vi "Wii Out.vi"(4 "error in":errorcluster, 6 "Calibration Data In":T6={"Wiimote 0G Calibration"={"Acceleration X"=127.0, "Acceleration Y"=131.0, "Acceleration Z"=126.0}, "Wiimote 1G Calibration"={"Acceleration X"=127.0, "Acceleration Y"=131.0, "Acceleration Z"=126.0}, "Nunchuk 0G Calibration"={"Acceleration X"=127.0, "Acceleration Y"=131.0, "Acceleration Z"=126.0}, "Nunchuk 1G Calibration"={"Acceleration X"=127.0, "Acceleration Y"=131.0, "Acceleration Z"=126.0}}, 7 "index":i32) -> (0 "error out":errorcluster, 2 "Wii output cluster":T5, 3 "hWiimoteHandle out":u32)   [LabVIEW 2011]
uses:
  Wiimote/Wiimote Buttons.ctl
  Wiimote/Nunchuk Buttons.ctl
  Wiimote/Wiimote Acceleration.ctl
  Wiimote/Wiimote Point.ctl
  Wiimote.lvlib
panel:
  in  "Offset":cluster{"X":dbl, "Y":dbl}={"X"=127.0, "Y"=127.0}
  out "Nunchuk Analog Stick":cluster{dbl, dbl}
  out "Nunchuk Analog Stick":cluster{dbl, dbl}[](graph)
  out "Nunchuk Acceleration":T7(graph)
  out "Wiimote Acceleration":T7(graph)
  out "Nunchuk Buttons":T4
  out "IR Sensor":cluster{"X":u16, "Y":u16}[](graph)
  out "Wiimote Buttons":T3
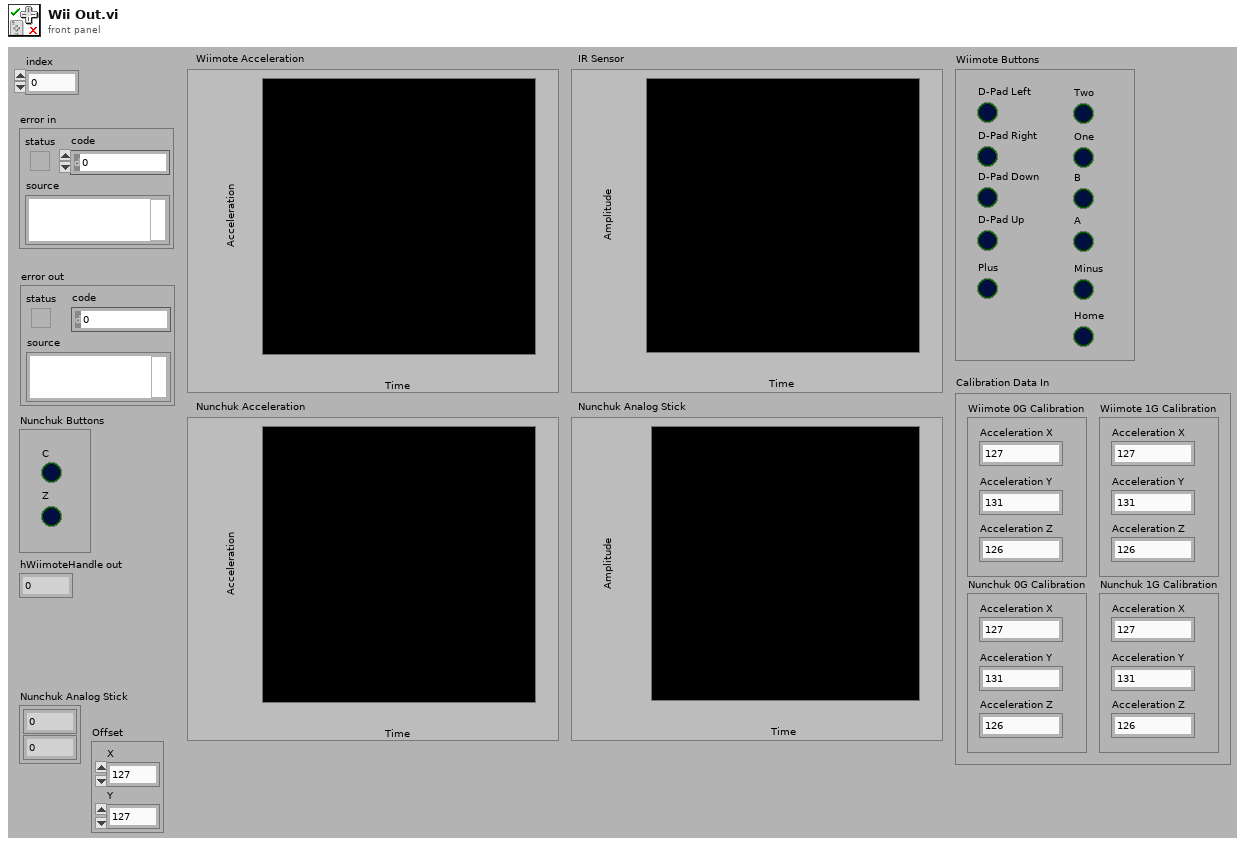
[diagram p1: front panel]
types:
  T1 = typedef "Wiimote.lvlib/Wiimote Acceleration.ctl" = cluster{"Acceleration X":dbl, "Acceleration Y":dbl, "Acceleration Z":dbl}
  T2 = typedef "Wiimote.lvlib/Wiimote Point.ctl" = cluster{"X":u16, "Y":u16}
  T3 = typedef "Wiimote.lvlib/Wiimote Buttons.ctl" = cluster{"D-Pad Left":bool, "D-Pad Right":bool, "D-Pad Down":bool, "D-Pad Up":bool, "Plus":bool, "Two":bool, "One":bool, "B":bool, "A":bool, "Minus":bool, "Home":bool}
  T4 = typedef "Wiimote.lvlib/Nunchuk Buttons.ctl" = cluster{"C":bool, "Z":bool}
  T5 = cluster{"Acceleration Calibrated Out":T1, "Acceleration Calibrated Out":T1, T2[], "Wiimote Buttons":T3, "Nunchuk Buttons":T4, "Nunchuk Analog Stick":cluster{"X":dbl, "Y":dbl}}
  T6 = cluster{"Wiimote 0G Calibration":T1, "Wiimote 1G Calibration":T1, "Nunchuk 0G Calibration":T1, "Nunchuk 1G Calibration":T1}
  T7 = cluster{"Acceleration X":dbl, "Acceleration Y":dbl, "Acceleration Z":dbl}
  T8 = typedef "Wiimote.lvlib/Wiimote IR Sensor.ctl" = cluster{"Point 1":T2, "Point 2":T2, "Point 3":T2, "Point 4":T2}
  T9 = cluster{"Wiimote Buttons":T3, "Wiimote Acceleration Raw":T1, "Wiimote IR Sensor":T8, "Nunchuk Analog Stick":T2, "Nunchuk Acceleration Raw":T1, "Nunchuk Buttons":T4}
  T10 = cluster{"Acceleration Calibrated Out":T1, "Acceleration Calibrated Out":T1, T2[], "Wiimote Buttons":T3, "Nunchuk Buttons":T4, cluster{"X":dbl, "Y":dbl}}
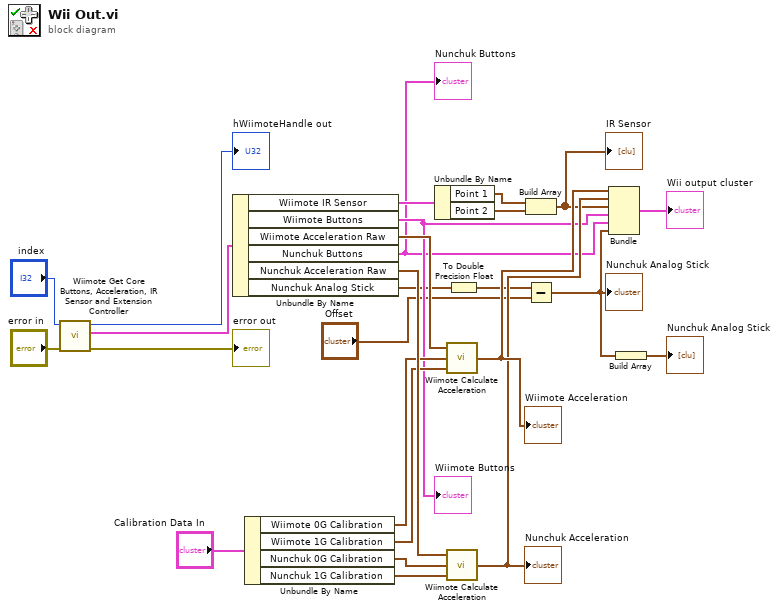
[diagram p0: block diagram]
diagram:
  n1 = call "Wiimote Get Core Buttons, Acceleration, IR Sensor and Extension Controller.vi"("error in"="error in", "hWiimoteHandle in"="index") -> ("error out"=→"error out":errorcluster, "Data out"=w21:T9, "hWiimoteHandle out"=→"hWiimoteHandle out":u32)  [unwired: 7 in]
  n2 = Unbundle By Name(w21) -> ("Wiimote IR Sensor"=w20:T8, "Wiimote Buttons"=w7:T3, "Wiimote Acceleration Raw"=w18:T1, "Nunchuk Buttons"=w6:T4, "Nunchuk Acceleration Raw"=w17:T1, "Nunchuk Analog Stick"=w5:T2)
  "Wiimote Buttons" <- w7
  "Nunchuk Buttons" <- w6
  n3 = Unbundle By Name("Calibration Data In") -> ("Wiimote 0G Calibration"=w13:T1, "Wiimote 1G Calibration"=w14:T1, "Nunchuk 0G Calibration"=w15:T1, "Nunchuk 1G Calibration"=w16:T1)
  n4 = Unbundle By Name(w20) -> ("Point 1"=w23:T2, "Point 2"=w22:T2)
  n5 = call "Wiimote Calculate Acceleration.vi"("Acceleration 1G Calibration"=w14, "Acceleration 0G Calibration"=w13, "Acceleration Raw in"=w18) -> ("Acceleration Calibrated Out"=w10:T1)
  "Wiimote Acceleration" <- w10
  n6 = call "Wiimote Calculate Acceleration.vi"("Acceleration 1G Calibration"=w16, "Acceleration 0G Calibration"=w15, "Acceleration Raw in"=w17) -> ("Acceleration Calibrated Out"=w9:T1)
  "Nunchuk Acceleration" <- w9
  n7 = To Double Precision Float(number=w5) -> (double precision float=w4:cluster{"X":dbl, "Y":dbl})
  n8 = Build Array(w23, w22) -> (w8:T2[])
  "IR Sensor" <- w8
  n9 = Subtract(x=w4, y="Offset") -> (x-y=w2:cluster{"X":dbl, "Y":dbl})
  "Nunchuk Analog Stick" <- w2
  n10 = Bundle("Acceleration Calibrated Out"=w10, "Acceleration Calibrated Out"=w9, w8, "Wiimote Buttons"=w7, "Nunchuk Buttons"=w6, w2) -> (→"Wii output cluster":T10)  [unwired: 1 in]
  n11 = Build Array(w2) -> (→"Nunchuk Analog Stick":cluster{"X":dbl, "Y":dbl}[])
